vi "Multi Folder Select.vi"(8 "error in":errorcluster, 11 "Root Folder Path":path caption="RM Data Folder Path:") -> (0 "error out":errorcluster, 3 "Tags":string[](array[string]))   [LabVIEW 2024]
uses:
  <vilib>/Utility/error.llb/DialogType.ctl
  Modules/Error handling/Controls/Error Command.ctl
  Modules/Error handling/Controls/Error Classification.ctl
  Modules/Tree Selection/Selection Global Method.ctl
panel:
  in  "Cancel Button 2":bool
  in  "OK Button":bool
  in  "Study Tree (live)":string[](tree)
  # "Select all images to analyse..."
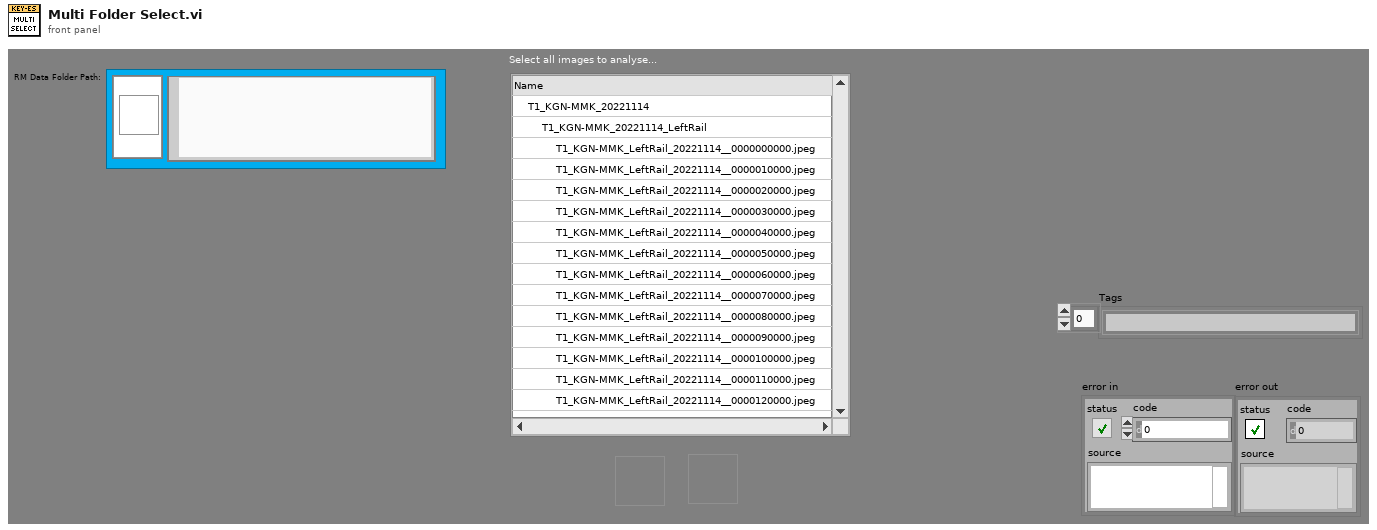
[diagram p1: front panel]
types:
  T1 = typedef "DialogType.ctl" = u16
  T2 = typedef "Error Classification.ctl" = enum16{"Warning", "Non-Critical", "Critical"}
  T3 = typedef "Error Command.ctl" = enum16{"Initialisation", "Handle", "Close"}
  T4 = typedef "LVPoint32TypeDef.ctl" = cluster{"Horizontal":i32, "Vertical":i32}
  T5 = typedef "Selection Global Method.ctl" = enum16{"Read Selection", "Force Selection", "Mouse Down Event", "Select All", "Select None", "Invert Selection", "Read Selection and Tags"}
  T6 = enum32{"invalid app kind", "Development System", "Run Time System", "Student Edition", "Embedded LabVIEW", "Evaluation", "Custom"}
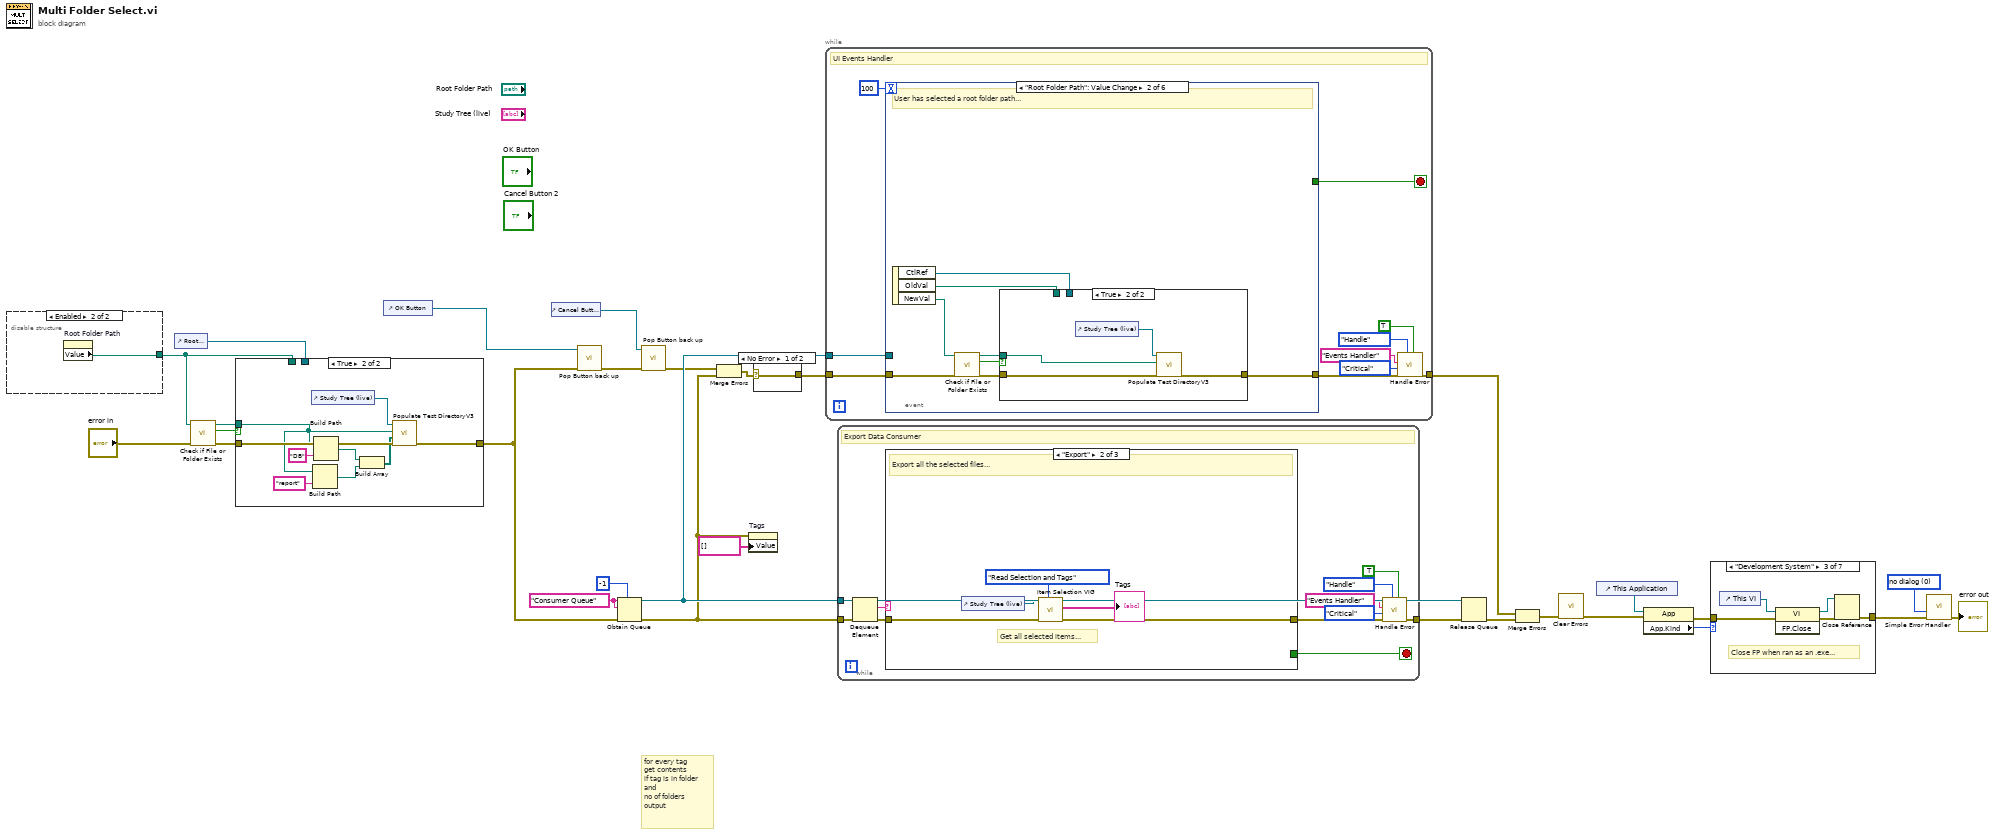
[diagram p0: block diagram]
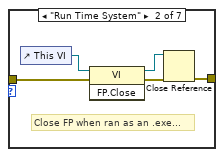
[diagram p3: hidden frame]
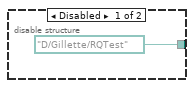
[diagram p8: hidden frame]
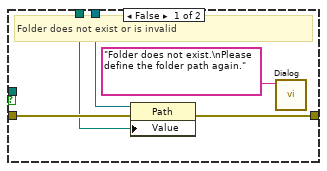
[diagram p9: hidden frame]
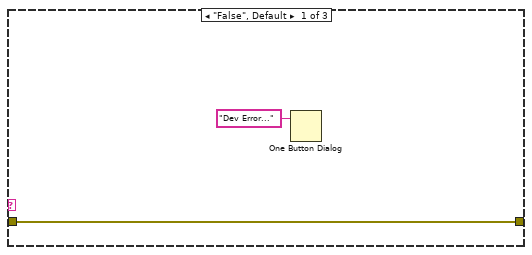
[diagram p11: hidden frame]
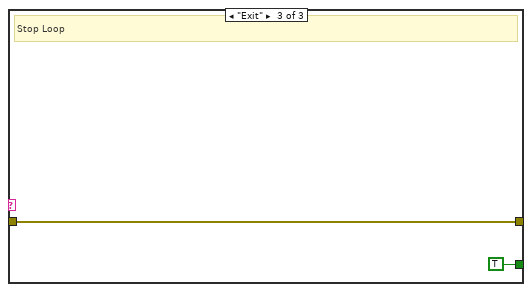
[diagram p12: hidden frame]
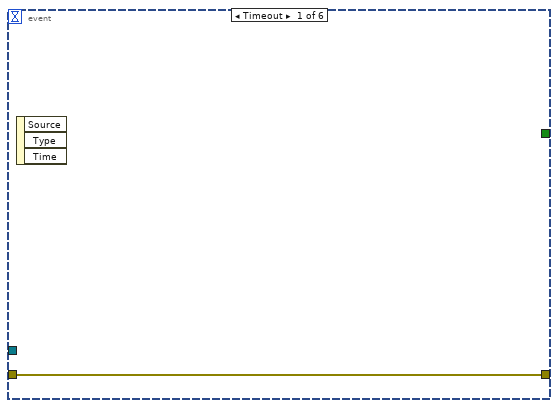
[diagram p13: hidden frame]
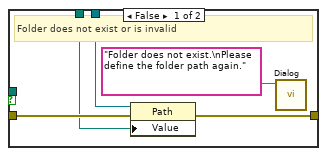
[diagram p14: hidden frame]
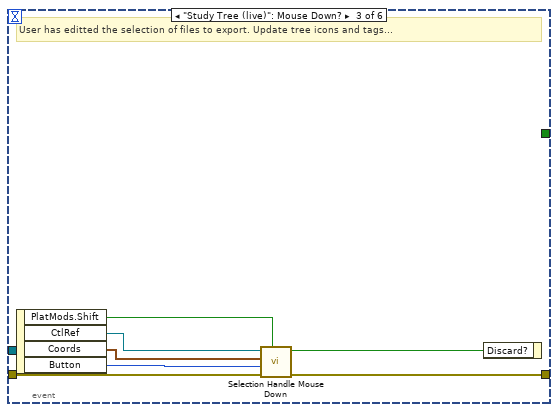
[diagram p15: hidden frame]
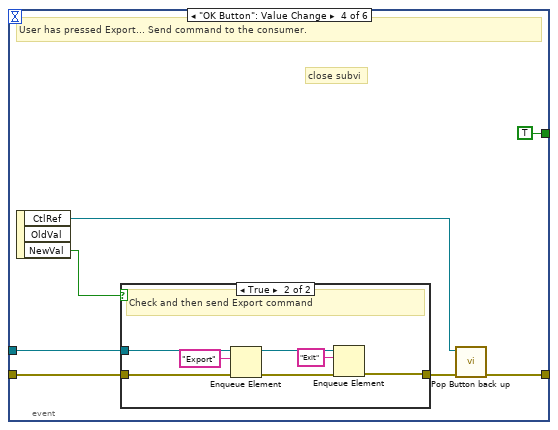
[diagram p16: hidden frame]
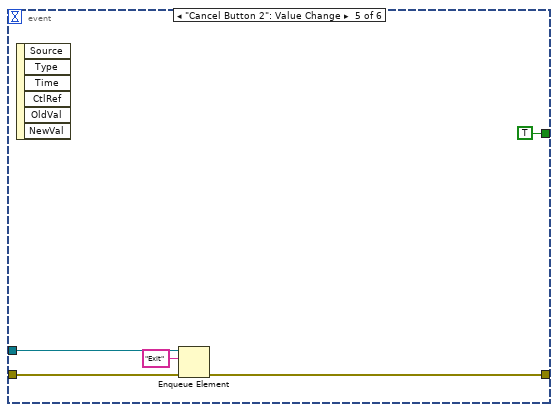
[diagram p18: hidden frame]
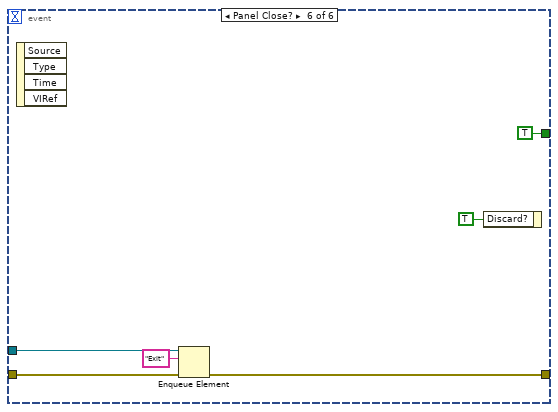
[diagram p19: hidden frame]
diagram:
  w21 = T1 0 items=["no dialog", "OK message", "continue or stop message", "OK message + warnings", "continue/stop + warnings"] ("type of dialog (OK msg:1)")
  w28 = "Consumer Queue" ("name (unnamed)")
  # "for every tag\nget contents\nif tag is in folder\nand\nno of folders\noutput"
  n1 = disable-structure shown="Enabled" {
    disable-tunnel: [path "D:/Gillette/RQTest" ("Value") w31] -> w5
    frame Disabled {
    }
    frame Enabled {
      n2 = property on="Root Folder Path" class="Path"() -> ("Value"=w31:path)  [unwired: 2 in, 2 out]
    }
  }
  n3 = control-ref of="Root Folder Path"() -> (w10:refnum<vi>)
  n4 = call <vilib>:"Check if File or Folder Exists.vi"("error in (no error)"="error in", "path"=w5) -> ("error out"=w11:errorcluster, "file or folder exists?"=w12:bool, "dup path"=w13:path)  [unwired: 7 in]
  n5 = case shown="True" w12 {
    tunnel: w10 -> [w36 _]
    tunnel: [w33 w44] -> w9
    tunnel: w11 -> [w35 w45]
    tunnel: w5 -> [w34 _]
    tunnel: w13 -> [_ w40]
    frame False {
      # "Folder does not exist or is invalid"
      n6 = property class="Path"(reference=w36, error in=w35, "Value"=w34) -> (error out=w33:errorcluster)  [unwired: 1 out]
      n7 = call "Dialog.vi"("Message"="Folder does not exist.\nPlease define the folder path again.") -> ()  [unwired: 10 in, 1 out]
    }
    frame True {
      n8 = control-ref of="Study Tree (live)"() -> (w43:refnum<vi>)
      n9 = Build Path(base path=w40, name or relative path="report") -> (appended path=w38:path)
      n10 = Build Path(base path=w40, name or relative path="DB") -> (appended path=w39:path)
      n11 = Build Array(w39, w38) -> (w37:path[])
      n12 = call "Populate Test DirectoryV3.vi"("error in (no error)"=w45, "FilePaths to Exclude"=w37, "Main Folder Path"=w40, "Study Tree (live)"=w43) -> ("error out"=w44:errorcluster)  [unwired: 7 in]
    }
  }
  n13 = control-ref of="OK Button"() -> (w4:refnum<vi>)
  n14 = control-ref of="Cancel Button 2"() -> (w2:refnum<vi>)
  n15 = call "Pop Button back up.vi"("error in (no error)"=w9, "Boolean in"=w4) -> ("error out"=w3:errorcluster)  [unwired: 9 in]
  n16 = Obtain Queue(max queue size (-1, unlimited)=-1, name (unnamed)=w28, element data type=w28, error in (no error)=w9) -> (queue out=w26:refnum<queue>, error out=w6:errorcluster)  [unwired: 1 in, 1 out]
  n17 = call "Pop Button back up.vi"("error in (no error)"=w3, "Boolean in"=w2) -> ("error out"=w1:errorcluster)  [unwired: 9 in]
  n18 = Merge Errors(w1, w6) -> (w16:errorcluster)
  n19 = property on="Tags" class="Arr (strict)"(error in=w6, "Value"=string[] []) -> ()  [unwired: 1 in, 2 out]
  n20 = case shown="No Error" w16 {
    selector: w16 -> [w46 _]
    tunnel: [w46 _] -> w15
    frame No Error {
    }
    frame Error {
    }
  }
  n21 = while {
    tunnel: w26 -> [w55]
    tunnel: w15 -> [w54]
    tunnel: [w52] -> w18
    stop <- w56 stop-if-true
    # "UI Events Handler"
    n22 = event shown="[1] \"Root Folder Path\": Value Change" {
      selector: _ -> [_ _ _ _ _ _]
      dyn-events: _ -> [_ _ _ _ _ _]
      timeout: 100 -> [_ _ _ _ _ _]
      tunnel: [_ _ _ TRUE TRUE TRUE] -> w56
      tunnel: w55 -> [_ _ _ w87 w99 w105]
      tunnel: w54 -> [w57 w63 w77 w88 w100 w106]
      tunnel: [w57 w64 w76 w86 w97 w102] -> w53
      event Timeout {
        n23 = event-data() -> ()  [unwired: 1 in, 3 out]
      }
      event "Root Folder Path": Value Change {
        # "User has selected a root folder path..."
        n24 = event-data() -> ("CtlRef"=w65:refnum<vi>, "OldVal"=w59:path, "NewVal"=w61:path)  [unwired: 1 in]
        n25 = call <vilib>:"Check if File or Folder Exists.vi"("error in (no error)"=w63, "path"=w61) -> ("error out"=w62:errorcluster, "file or folder exists?"=w60:bool, "dup path"=w58:path)  [unwired: 7 in]
        n26 = case shown="True" w60 {
          tunnel: w65 -> [w70 _]
          tunnel: [w67 w73] -> w64
          tunnel: w62 -> [w69 w74]
          tunnel: w59 -> [w68 _]
          tunnel: w58 -> [_ w72]
          frame False {
            # "Folder does not exist or is invalid"
            n27 = property class="Path"(reference=w70, error in=w69, "Value"=w68) -> (error out=w67:errorcluster)  [unwired: 1 out]
            n28 = call "Dialog.vi"("Message"="Folder does not exist.\nPlease define the folder path again.") -> ()  [unwired: 10 in, 1 out]
          }
          frame True {
            n29 = control-ref of="Study Tree (live)"() -> (w71:refnum<vi>)
            n30 = call "Populate Test DirectoryV3.vi"("error in (no error)"=w74, "Main Folder Path"=w72, "Study Tree (live)"=w71) -> ("error out"=w73:errorcluster)  [unwired: 8 in]
          }
        }
      }
      event "Study Tree (live)": Mouse Down? {
        # "User has editted the selection of files to export. Update tree icons and tags..."
        n31 = event-data() -> ("PlatMods.Shift"=w78:bool, "CtlRef"=w79:refnum<vi>, "Coords"=w81:T4, "Button"=w80:u16)  [unwired: 1 in]
        n32 = call "Selection Handle Mouse Down.vi"("Shift?"=w78, "error in (no error)"=w77, "Mouse Button"=w80, "Mouse Coords"=w81, "Listbox or Tree"=w79) -> ("error out"=w76:errorcluster, "Discard?"=w75:bool)  [unwired: 5 in]
        n33 = event-data("Discard?"=w75) -> ()  [unwired: 1 in, 1 out]
      }
      event "OK Button": Value Change {
        # "close subvi"
        # "User has pressed Export... Send command to the consumer."
        n34 = event-data() -> ("CtlRef"=w85:refnum<vi>, "NewVal"=w82:bool)  [unwired: 1 in, 1 out]
        n35 = case shown="True" w82 {
          tunnel: w88 -> [w89 w95]
          tunnel: [w89 w90] -> w83
          tunnel: w87 -> [_ w96]
          frame False {
            # "Do nothing..."
          }
          frame True {
            # "Check and then send Export command"
            n36 = Enqueue Element(queue=w96, element="Export", error in (no error)=w95) -> (queue out=w92:refnum<queue>, error out=w91:errorcluster)  [unwired: 1 in, 1 out]
            n37 = Enqueue Element(queue=w92, element="Exit", error in (no error)=w91) -> (error out=w90:errorcluster)  [unwired: 1 in, 2 out]
          }
        }
        n38 = call "Pop Button back up.vi"("error in (no error)"=w83, "Boolean in"=w85) -> ("error out"=w86:errorcluster)  [unwired: 9 in]
      }
      event "Cancel Button 2": Value Change {
        n39 = event-data() -> ()  [unwired: 1 in, 6 out]
        n40 = Enqueue Element(queue=w99, element="Exit", error in (no error)=w100) -> (error out=w97:errorcluster)  [unwired: 1 in, 2 out]
      }
      event Panel Close? {
        n41 = event-data() -> ()  [unwired: 1 in, 4 out]
        n42 = Enqueue Element(queue=w105, element="Exit", error in (no error)=w106) -> (error out=w102:errorcluster)  [unwired: 1 in, 2 out]
        n43 = event-data("Discard?"=TRUE) -> ()  [unwired: 1 in, 1 out]
      }
    }
    n44 = call "Handle Error.vi"("Clear Error?"=TRUE, "Command"=Error_Command."Handle", "error in (no error)"=w53, "Classification"=Error_Classification."Critical", "Section of Code"="Events Handler" ("Test Name")) -> ("error out"=w52:errorcluster)  [unwired: 4 in, 2 out]
  }
  n45 = while {
    tunnel: w26 -> [w118]
    tunnel: w6 -> [w117]
    tunnel: [w108] -> w29
    stop <- w114 stop-if-true
    # "Export Data Consumer"
    n46 = Dequeue Element(queue=w118, error in (no error)=w117) -> (element=w115:string, error out=w116:errorcluster)  [unwired: 1 in, 2 out]
    n47 = case shown="\"Export\"" w115 {
      tunnel: [w120 w121 w127] -> w109
      tunnel: w116 -> [w120 w124 w127]
      tunnel: [_ _ TRUE] -> w114
      frame "False", Default {
        n48 = One Button Dialog(message="Dev Error...") -> ()  [unwired: 1 in, 1 out]
      }
      frame "Export" {
        # "Get all selected items..."
        # "Export all the selected files..."
        n49 = control-ref of="Study Tree (live)"() -> (w123:refnum<vi>)
        n50 = call "Item Selection VIG.vi"("Method (Read Selection)"=Selection_Global_Method."Read Selection and Tags", "error in (no error)"=w124, "Listbox or Tree"=w123) -> ("error out"=w121:errorcluster, "Tags"=→"Tags":string[])  [unwired: 6 in, 1 out]
      }
      frame "Exit" {
        # "Stop Loop"
      }
    }
    n51 = call "Handle Error.vi"("Clear Error?"=TRUE, "Command"=Error_Command."Handle", "error in (no error)"=w109, "Classification"=Error_Classification."Critical", "Section of Code"="Events Handler" ("Test Name")) -> ("error out"=w108:errorcluster)  [unwired: 4 in, 2 out]
  }
  n52 = Release Queue(queue=w26, error in (no error)=w29) -> (error out=w20:errorcluster)  [unwired: 1 in, 2 out]
  n53 = Merge Errors(w18, w20) -> (w19:errorcluster)
  n54 = call <vilib>:"Clear Errors.vi"("error in (no error)"=w19) -> ("error out"=w17:errorcluster)  [unwired: 5 in, 1 out]
  n55 = control-ref of="This Application"() -> (w23:refnum<vi>)
  n56 = property class="App"(reference=w23, error in=w17) -> (error out=w25:errorcluster, "App.Kind"=w24:T6)  [unwired: 1 out]
  n57 = case shown="\"Development System\"" w24 {
    tunnel: w25 -> [w128 w132 w137 w139 w140 w141 w142]
    tunnel: [w128 w129 w134 w139 w140 w141 w142] -> w22
    frame "invalid app kind", Default {
    }
    frame "Run Time System" {
      # "Close FP when ran as an .exe..."
      n58 = control-ref of="This VI"() -> (w133:refnum<vi>)
      n59 = invoke class="VI" method="FP.Close"(reference=w133, error in=w132) -> (reference out=w130:refnum<vi>, error out=w131:errorcluster)  [unwired: 1 in, 1 out]
      n60 = Close Reference(reference=w130, error in (no error)=w131) -> (error out=w129:errorcluster)
    }
    frame "Development System" {
      # "Close FP when ran as an .exe..."
      n61 = control-ref of="This VI"() -> (w138:refnum<vi>)
      n62 = invoke class="VI" method="FP.Close"(reference=w138, error in=w137) -> (reference out=w135:refnum<vi>, error out=w136:errorcluster)  [unwired: 1 in, 1 out]
      n63 = Close Reference(reference=w135, error in (no error)=w136) -> (error out=w134:errorcluster)
    }
    frame "Student Edition" {
    }
    frame "Embedded LabVIEW" {
    }
    frame "Evaluation" {
    }
    frame "Custom" {
    }
  }
  n64 = call <vilib>:"Simple Error Handler.vi"("type of dialog (OK msg:1)"=w21, "error in (no error)"=w22) -> ("error out"=→"error out":errorcluster)  [unwired: 3 in, 4 out]
